vi "Init Data.vi"(8 "error in (no error)":errorcluster, 11 "Rigol DG822 Sine in":refnum<class "Rigol DG822 Sine.lvclass">) -> (0 "error out":errorcluster, 3 "Rigol DG822 Sine out":refnum<class "Rigol DG822 Sine.lvclass">)   [LabVIEW 2021, in "Rigol DG822 UI.lvlib" / "Rigol DG822 Sine.lvlib" / "Rigol DG822 Sine.lvclass"]
uses:
  Rigol DG822 Sine.lvclass
  Rigol DG822 Sine.lvclass/Rigol DG822 Sine.ctl
  General/Files/lvlibp/Actors.lvlibp/Actors/Actors/Actors.lvclass
  D:/LabVIEW/General/Files/lvlibp/Actors.lvlibp/Actors/Actors/Actors.lvclass
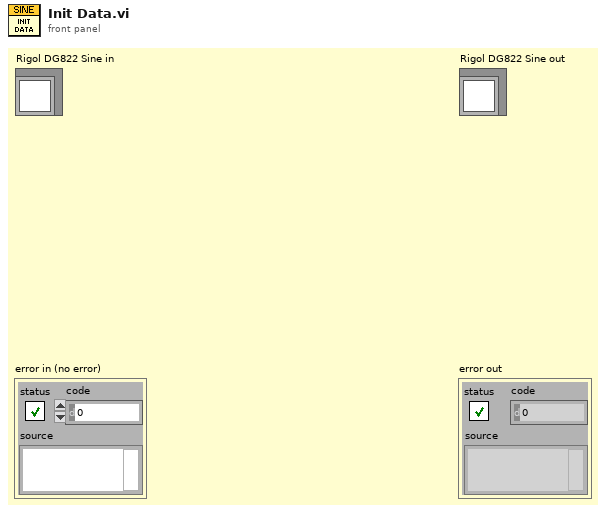
[diagram p1: front panel]
types:
  T1 = cluster{"Freq-Period":string, "Freq-Period 2":string, "Freq-Period 3":string, "Freq-Period 4":string}
  T2 = cluster{"Control Label":string, "Control Label 2":string, "Control Label 3":string}
  T3 = cluster{"Control Label 5":string, "Control Label 6":string, "Control Label":string, "Control Label 2":string, "Control Label 3":string, "Control Label 4":string}
  T4 = typedef "FT Controls Cluster.ctl" = cluster{"Freq/Period":bool, "Ampl/HighL":bool, "Offset/LowL":bool, "Duty/Width":bool}
  T5 = typedef "String Indicators Cluster.ctl" = cluster{"Freq-Period":string, "Ampl-HighL":string, "Offset-LowL":string, "Phase":string, "Duty-Width":string, "RisEdge":string, "FallEdge":string}
  T6 = enum32{"No Selection", "MHz", "kHz", "Hz", "mHz", "uHz"}
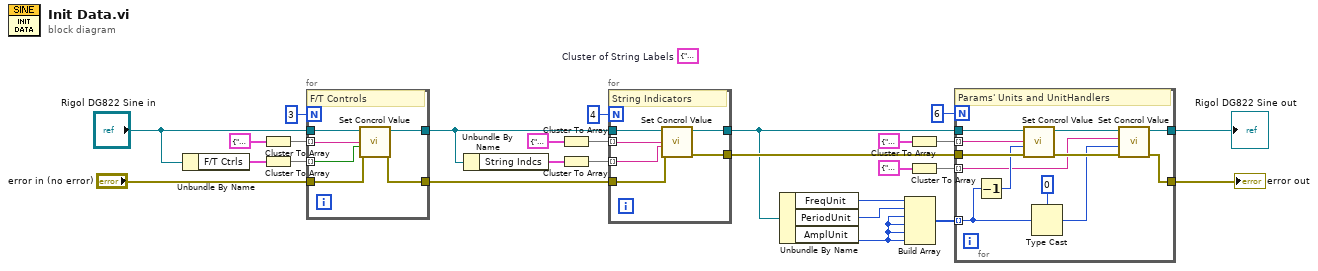
[diagram p0: block diagram]
diagram:
  (unwired) T1 {"Freq-Period"="String Indcs.Freq-Period", "Freq-Period 2"="String Indcs.Ampl-HighL", "Freq-Period 3"="String Indcs.Offset-LowL", "Freq-Period 4"="String Indcs.Phase"}  # Cluster of String Labels
  n1 = Unbundle By Name("Rigol DG822 Sine in") -> ("F/T Ctrls"=w22:T4)
  n2 = Cluster To Array(cluster=T2 {"Control Label"="F/T Ctrls.Freq/Period", "Control Label 2"="F/T Ctrls.Ampl/HighL", "Control Label 3"="F/T Ctrls.Offset/LowL"}) -> (array=w20:string[])
  n3 = Cluster To Array(cluster=w22) -> (array=w18:bool[])
  n4 = for {
    N: 3 -> [_]
    tunnel: w20 -> [w33] mode=indexing
    tunnel: "Rigol DG822 Sine in" -> [w32]
    tunnel: w18 -> [w31] mode=indexing
    tunnel: "error in (no error)" -> [w30]
    tunnel: [w29] -> w14
    tunnel: [w28] -> w10
    # "F/T Controls"
    n5 = call "Set Concrol Value.vi"("error in (no error)"=w30, "Value"=w31, "Control Label"=w33, "Actors in"=w32) -> ("error out"=w29:errorcluster, "Actors out"=w28:refnum<class "Rigol DG822 Sine.lvclass">)  [unwired: 6 in]
  }
  n6 = Unbundle By Name(w10) -> ("String Indcs"=w13:T5)
  n7 = Cluster To Array(cluster=T1 {"Freq-Period"="String Indcs.Freq-Period", "Freq-Period 2"="String Indcs.Ampl-HighL", "Freq-Period 3"="String Indcs.Offset-LowL", "Freq-Period 4"="String Indcs.Phase"} ("Cluster of String Labels")) -> (array=w11:string[])
  n8 = Cluster To Array(cluster=w13) -> (array=w12:string[])
  n9 = for {
    N: 4 -> [_]
    tunnel: w11 -> [w39] mode=indexing
    tunnel: w10 -> [w38]
    tunnel: w12 -> [w37] mode=indexing
    tunnel: w14 -> [w36]
    tunnel: [w35] -> w8
    tunnel: [w34] -> w6
    # "String Indicators"
    n10 = call "Set Concrol Value.vi"("error in (no error)"=w36, "Value"=w37, "Control Label"=w39, "Actors in"=w38) -> ("error out"=w35:errorcluster, "Actors out"=w34:refnum<class "Rigol DG822 Sine.lvclass">)  [unwired: 6 in]
  }
  n11 = Unbundle By Name(w6) -> ("FreqUnit"=w5:T6, "PeriodUnit"=w3:enum32{"No Selection", "s", "ms", "us", "ns"}, "AmplUnit"=w4:enum32{"No Selection", "Vpp", "mVpp"})
  n12 = Build Array(w5, w3, w4, w4, w4, w4) -> (w7:u32[])
  n13 = Cluster To Array(cluster=T3 {"Control Label 5"="FreqUnitHandler", "Control Label 6"="PeriodUnitHandler", "Control Label"="AmplUnitHandler", "Control Label 2"="HighLUnitHandler", "Control Label 3"="OffsetUnitHandler", "Control Label 4"="LowLUnitHandler"}) -> (array=w25:string[])
  n14 = Cluster To Array(cluster=T3 {"Control Label 5"="FreqUnit", "Control Label 6"="PeriodUnit", "Control Label"="AmplUnit", "Control Label 2"="HighLUnit", "Control Label 3"="OffsetUnit", "Control Label 4"="LowLUnit"}) -> (array=w23:string[])
  n15 = for {
    N: 6 -> [_]
    tunnel: w6 -> [w50]
    tunnel: [w48] -> w2
    tunnel: [w47] -> w1
    tunnel: w8 -> [w46]
    tunnel: w25 -> [w45] mode=indexing
    tunnel: w23 -> [w43] mode=indexing
    tunnel: w7 -> [w40] mode=indexing
    # "Params' Units and UnitHandlers"
    n16 = Decrement(x=w40) -> (x-1=w44:u32)
    n17 = call "Set Concrol Value.vi"("error in (no error)"=w46, "Value"=w44, "Control Label"=w45, "Actors in"=w50) -> ("error out"=w51:errorcluster, "Actors out"=w49:refnum<class "Rigol DG822 Sine.lvclass">)  [unwired: 6 in]
    n18 = Type Cast(type=0, x=w40) -> (*(type *) &x=w42:i32)
    n19 = call "Set Concrol Value.vi"("error in (no error)"=w51, "Value"=w42, "Control Label"=w43, "Actors in"=w49) -> ("error out"=w47:errorcluster, "Actors out"=w48:refnum<class "Rigol DG822 Sine.lvclass">)  [unwired: 6 in]
  }
  "error out" <- w1
  "Rigol DG822 Sine out" <- w2
